vi "Global ROTORE BLOCCATO SETTINGS.vi"() -> ()   [LabVIEW 2019]
uses:
  TypeDef/Control rotore bloccato.ctl
panel:
  in  "Rotore bloccato":T1={"TEMPO PROVA"=0.1} {"TEMPO PROVA" min=0.1 format="%#.1f s"}
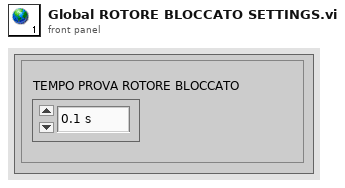
[diagram p1: front panel]
types:
  T1 = typedef "Control rotore bloccato.ctl" = cluster{"TEMPO PROVA":dbl}
diagram:
